vi "Vision Update Time.vi"   [LabVIEW 2023]
uses:
  <vilib>/Rock Robotics/Network Tables/NT Write Number.vi
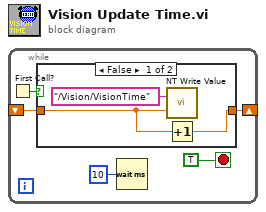
[diagram p0: block diagram]
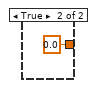
[diagram p2: hidden frame]
diagram:
  n1 = while {
    shift-right: [w2] -> _
    shift-left: _ -> [w3]
    stop <- TRUE stop-if-true
    n2 = First Call?() -> (First Call?: T/F=w4:bool)
    n3 = case shown="False" w4 {
      tunnel: w3 -> [w7 _]
      tunnel: [w6 0.0] -> w2
      frame False {
        n4 = call-poly <vilib>:"NT Write Value.vi"("value"=w7, "name"="/Vision/VisionTime" ("Name")) -> ()  [unwired: 9 in, 1 out]
        n5 = Increment(x=w7) -> (x+1=w6:dbl)
      }
      frame True {
      }
    }
    n6 = Wait (ms)(milliseconds to wait=u32 10) -> ()  [unwired: 1 out]
  }
